vi "SCMP - Run Cookbook.vi"(0 "Cookbook":T13=[{"Data Type"=enum."SET EXPOSURE", "Arg 1"=0.1, "Arg 2"=999.0, "Arg 3"=path "C:/SCD Cookbooks/exposure-100ms.rcp", "Comments"=""}, {"Data Type"=enum."ACQUIRE DATA", "Arg 1"=1.0, "Arg 2"=1.0, "Arg 3"=path "C:/SCD Cookbooks/aaa.rcp", "Comments"=""}], 1 "Mod/Seq":bool, 3 "Save to FITS?":bool=TRUE, 5 "limit max FPS to:":dbl=20.0 format="%0.2p", 7 "Motors":bool=TRUE, 11 "Error in":errorcluster, 12 "Andor Neo":T1[](array[typedef]) {"Exposure (s)" format="%^.3g"; "Time at Synch" format="%<%H:%M:%S>T"; "Interframe Time" format="%#_3g"; "Frame Readout Time" format="%_3g"; "Row Readout Time" format="%_3g"}, 13 "FITS Header In":T4={"Wavelength (nm)"=530.15, "Exposure (s)"=0.05, "Tuning Delay (ms)"=1000.0, "Beam Type (-1/1)"=1.0, "Tuning Voltages"=[1.111, 2.222, 3.333, 4.444], "Observer"="observer", "Light Shapping Diffuser"=enum."In Beam", "Comment"="", "Data Type"=9, "Mod Cycles"=0, "SCD Calibration Optics"=enum."1 - Polarizer @0, I+Q", "SCD Emission Line Filter"=enum."1-557.6nm", "Cookbook"="", "COMP-S Calibration Wheel"=enum."Dark", "COMP-S Andover Filter Wheel"=enum."530.3nm/HWB 0.34nm (Fe XIV)", "FOV Rotation (deg)"=66.0, "Objective Lens Position (mm)"=0.0, "Occulter size"=0.0, "Time End"=timestamp(3382374145.421875 s since 1904-01-01), "Acc Exposure (s)"=0.0, "Time Stamp Array"=[], "Camera Serial Number"=[], "Camera Temp"=[], "Camera PI (mm)"=[], "Time Start"=timestamp(3382374145.421875 s since 1904-01-01), "Peripherals"={"ILX controler"=FALSE, "Zone temperatures"=FALSE, "Andor"=FALSE, "Andor 2"=FALSE, "PI Stages"=FALSE, "AISAS mechanisms"=FALSE, "AISAS Mech.lvclass"=refnum, "Zone temp ref"=variant, "FWs"=FALSE}, "FITS paths"=[], "Cameras"=enum."Andor", "load preset cbk"=FALSE, "periodic check count"=0} {"Camera PI (mm)" format="%_3g"; "Acc Exposure (s)" format="%^.3g"; "Occulter size" format="%.2f"; "Objective Lens Position (mm)" min=70.0 max=152.0 format="%.2f"; "FOV Rotation (deg)" format="%.1f"; "Data Type" items=["LIVE", "DARK", "FLAT", "CALI", "OBSE", "ABSO", "AURE", "TARG", "OBJE", "HOLE", "OREX", "THRO", "CHIP"]; "Exposure (s)" format="%^.3g"; "Wavelength (nm)" format="%_6g"}) -> (4 "Result":string, 6 "FITS Path Out":path, 14 "Updated Header":T4={"Wavelength (nm)"=530.15, "Exposure (s)"=0.05, "Tuning Delay (ms)"=1000.0, "Beam Type (-1/1)"=1.0, "Tuning Voltages"=[1.111, 2.222, 3.333, 4.444], "Observer"="observer", "Light Shapping Diffuser"=enum."In Beam", "Comment"="", "Data Type"=9, "Mod Cycles"=0, "SCD Calibration Optics"=enum."1 - Polarizer @0, I+Q", "SCD Emission Line Filter"=enum."1-557.6nm", "Cookbook"="", "COMP-S Calibration Wheel"=enum."Dark", "COMP-S Andover Filter Wheel"=enum."530.3nm/HWB 0.34nm (Fe XIV)", "FOV Rotation (deg)"=66.0, "Objective Lens Position (mm)"=0.0, "Occulter size"=0.0, "Time End"=timestamp(3382374145.421875 s since 1904-01-01), "Acc Exposure (s)"=0.0, "Time Stamp Array"=[], "Camera Serial Number"=[], "Camera Temp"=[], "Camera PI (mm)"=[], "Time Start"=timestamp(3382374145.421875 s since 1904-01-01), "Peripherals"={"ILX controler"=FALSE, "Zone temperatures"=FALSE, "Andor"=FALSE, "Andor 2"=FALSE, "PI Stages"=FALSE, "AISAS mechanisms"=FALSE, "AISAS Mech.lvclass"=refnum, "Zone temp ref"=variant, "FWs"=FALSE}, "FITS paths"=[], "Cameras"=enum."Andor", "load preset cbk"=FALSE, "periodic check count"=0} {"Camera PI (mm)" format="%_3g"; "Acc Exposure (s)" format="%^.3g"; "Occulter size" format="%.2f"; "Objective Lens Position (mm)" min=70.0 max=152.0 format="%.2f"; "FOV Rotation (deg)" format="%.1f"; "Data Type" items=["LIVE", "DARK", "FLAT", "CALI", "OBSE", "ABSO", "AURE", "TARG", "OBJE", "HOLE", "OREX", "THRO", "CHIP"]; "Exposure (s)" format="%^.3g"; "Wavelength (nm)" format="%_6g"}, 15 "Error out":errorcluster)   [LabVIEW 2014]
doc: "Use this template to build a VI to use as a subVI."
uses:
  Controls/Cookbook.ctl
  Controls/Cbk Data type.ctl
  Controls/SCD - FITS Cluster.ctl
  AISAS/Mech/AISAS Mech.lvclass
  AISAS/Controls/Diffuser.ctl
  Controls/SCD - Calibration Optics Filter Wheel.ctl
  Controls/SCD - EDT - Emission Line Filter Wheel.ctl
  Controls/CoMP-S Controls/Polarization Optics Filter Wheel.ctl
  Controls/CoMP-S Controls/Emission Line Filter Wheel.ctl
  AISAS/Controls/focus.ctl
  Controls/peripherals.ctl
  Controls/Cameras select.ctl
  Camera/Andor Neo Info.ctl
  Controls/beaning.ctl
  AISAS/Controls/motor.ctl
  AISAS/Mech/AISAS Mech.lvclass/AISAS Mech.ctl
  Controls/Globals.vi
  <vilib>/Utility/file.llb/Read From Spreadsheet File (DBL).vi
panel:
  out "Changes 0 or 1 to true/false for absolute or relative control 4":bool[](array[boolean])
  out "Changes 0 or 1 to true/false for absolute or relative control 3":bool[](array[boolean])
  out "rcp first row":dbl[](array[numeric]) format="%0.4f"
  out "Changes 0 or 1 to true/false for absolute or relative control 2":bool[](array[boolean])
  in  "Stop Cookbook":bool
  out "Recipe Being Processed":string
  out "Most Recent Image Accumulation (Modulation State A)":u32[][](graph)
  out "Headers Out":T4[](array[typedef]) {"Camera PI (mm)" format="%_3g"; "Acc Exposure (s)" format="%^.3g"; "Occulter size" format="%.2f"; "Objective Lens Position (mm)" min=70.0 max=152.0 format="%.2f"; "FOV Rotation (deg)" format="%.1f"; "Data Type" items=["LIVE", "DARK", "FLAT", "CALI", "OBSE", "ABSO", "AURE", "TARG", "OBJE", "HOLE", "OREX", "THRO", "CHIP"]; "Exposure (s)" format="%^.3g"; "Wavelength (nm)" format="%_6g"}
  out "LCVR Voltages":dbl[][](array[numeric]) format="%.4f"
  out "Total Recipes":i32=2
  out "Recipe Step":i32=1
  out "Mod Cycles":u16=1
  out "Exposure (s)":sgl=0.1
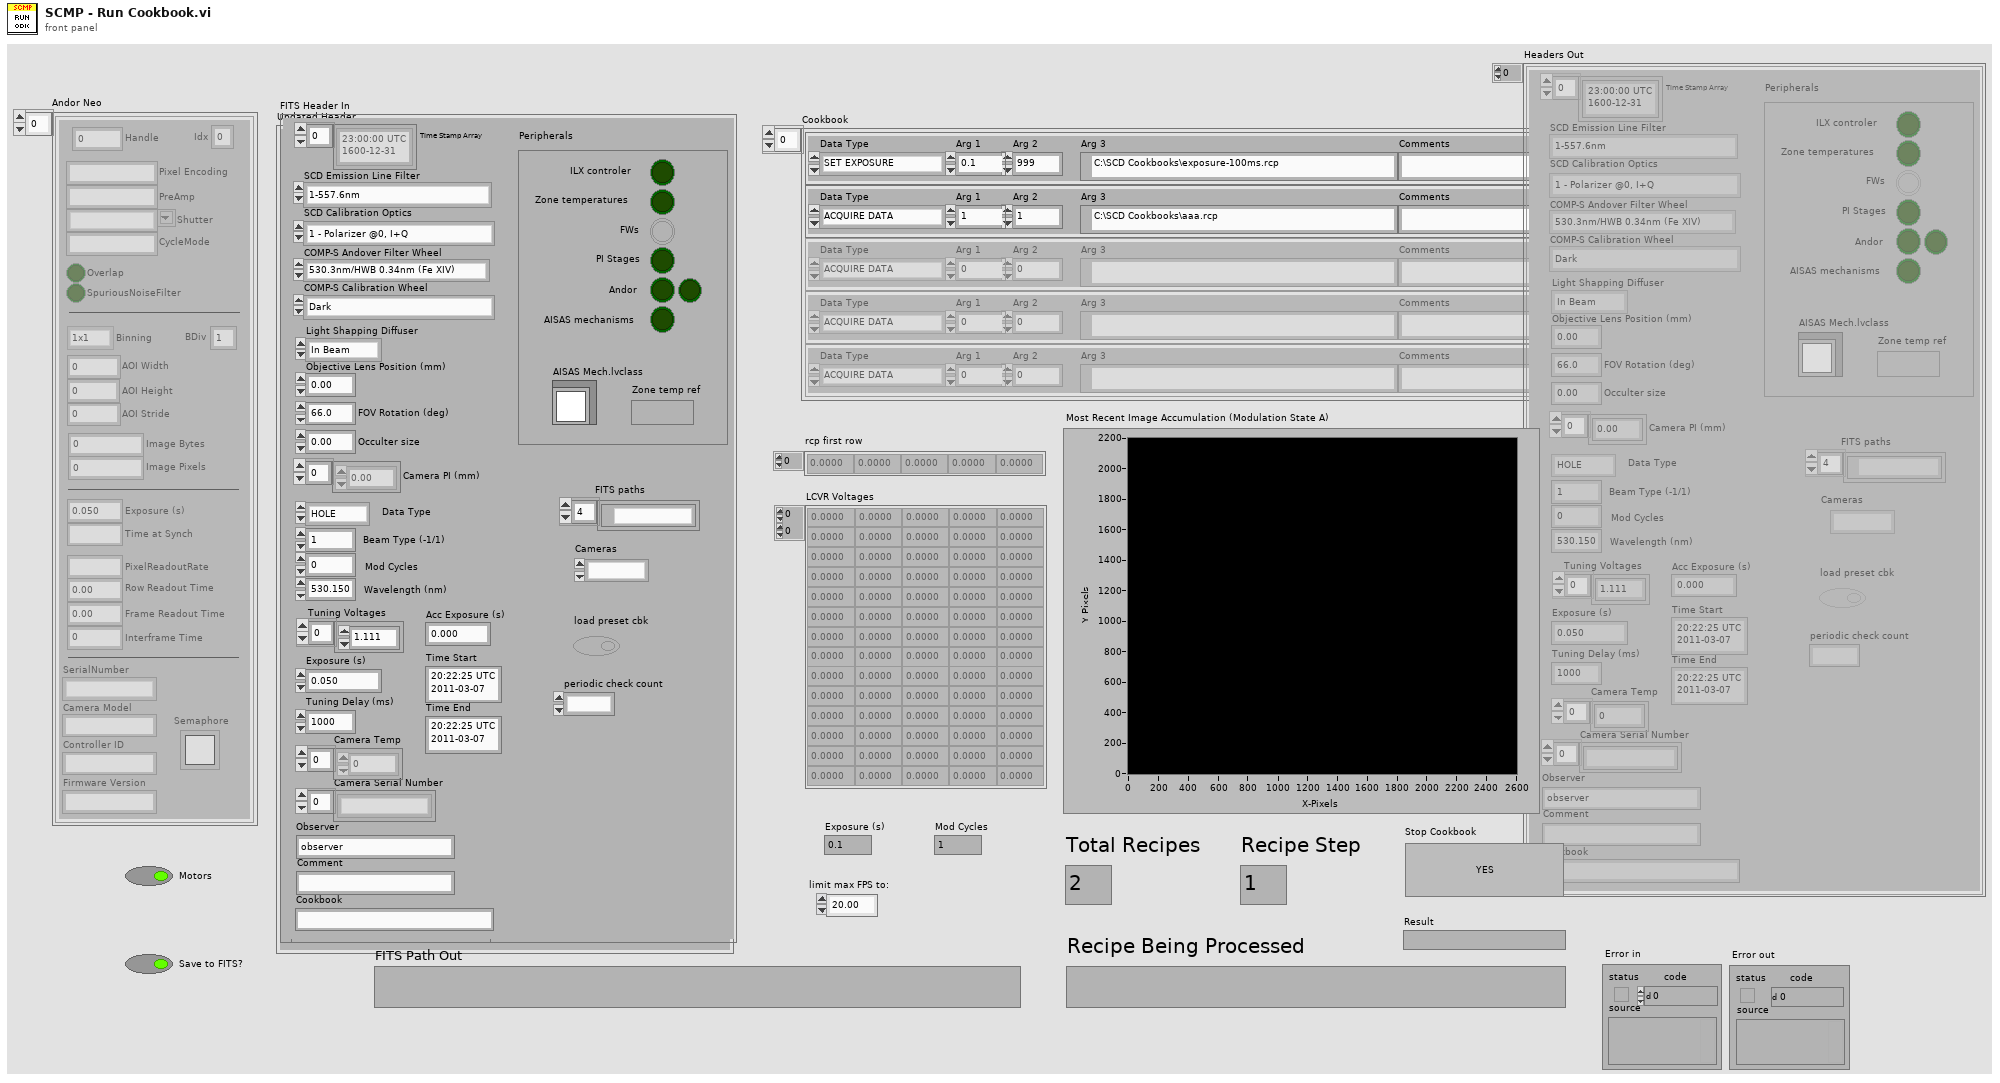
[diagram p1: front panel]
types:
  T1 = typedef "Andor Neo Info.ctl" = cluster{"Handle":i32, "Pixel Encoding":string, "AOI Width":i32, "AOI Height":i32, "AOI Stride":i32, "Row Readout Time":dbl, "Frame Readout Time":dbl, "Interframe Time":dbl, "Semaphore":T2, "SerialNumber":string, "Camera Model":string, "Controller ID":string, "Firmware Version":string, "Shutter":string, "BDiv":u8, "Time at Synch":timestamp, "Idx":i32, "PreAmp":string, "Binning":T3, "PixelReadoutRate":string, "Exposure (s)":dbl, "Image Bytes":i64, "Image Pixels":i64, "SpuriousNoiseFilter":bool, "Overlap":bool, "CycleMode":string}
  T2 = typedef "Semaphore RefNum" = refnum<k1>
  T3 = typedef "beaning.ctl" = enum16{"1x1", "2x2", "3x3", "4x4", "8x8"}
  T4 = typedef "SCD - FITS Cluster.ctl" = cluster{"Wavelength (nm)":dbl, "Exposure (s)":dbl, "Tuning Delay (ms)":dbl, "Beam Type (-1/1)":dbl, "Tuning Voltages":dbl[], "Observer":string, "Light Shapping Diffuser":T5, "Comment":string, "Data Type":u16, "Mod Cycles":u16, "SCD Calibration Optics":T6, "SCD Emission Line Filter":T7, "Cookbook":string, "COMP-S Calibration Wheel":T8, "COMP-S Andover Filter Wheel":T9, "FOV Rotation (deg)":dbl, "Objective Lens Position (mm)":T10, "Occulter size":dbl, "Time End":timestamp, "Acc Exposure (s)":dbl, "Time Stamp Array":timestamp[], "Camera Serial Number":string[], "Camera Temp":dbl[], "Camera PI (mm)":dbl[], "Time Start":timestamp, "Peripherals":T11, "FITS paths":path[], "Cameras":T12, "load preset cbk":bool, "periodic check count":i32}
  T5 = typedef "Diffuser.ctl" = enum16{"Out of Beam", "In Beam"}
  T6 = typedef "SCD - Calibration Optics Filter Wheel.ctl" = enum16{"1 - Polarizer @0, I+Q", "2 - Polarizer @90, I-Q", "3 - Polarizer @45, I+U", "4 - Polarizer @135, I-U", "5 - Polarizer @0, Retarder @45, I+V", "6 - Polarizer @0, Retarder @135, I-V", "7 - Dark", "8 - Clear", "9 - N/A"}
  T7 = typedef "SCD - EDT - Emission Line Filter Wheel.ctl" = enum16{"1-557.6nm", "2-587.6nm", "3-589.6nm", "4-630.2nm", "5-656.4nm", "6-849.8nm", "7-854.2nm", "8-866.2nm", "9-1083.0nm"}
  T8 = typedef "Polarization Optics Filter Wheel.ctl" = enum16{"Dark", "Clear", "Exchange Lens", "Polarizer @0, I+Q", "Polarizer @90, I-Q", "Polarizer @45, I+U", "Polarizer @135, I-U", "Polarizer @0, Retarder @45, I+V", "Polarizer @0, Retarder @135, I-V"}
  T9 = typedef "Emission Line Filter Wheel.ctl" = enum16{"530.3nm/HWB 0.34nm (Fe XIV)", "587.6nm/HBW 0.44nm (He I D3)", "637.5nm/HBW 0.53nm (Fe X)", "656.3nm/HBW 0.57nm (H-Alpha)", "789.2nm/HBW 0.85nm (Fe XI)", "854.2nm/HBW 1.01nm (Ca I)", "1074.7nm/HBW 2.34nm (Fe XIII)", "1079.8nm/HBW 1.64nm (Fe XIII)", "1083.0nm/HBW 1.66nm (He I)"}
  T10 = typedef "focus.ctl" = dbl
  T11 = typedef "peripherals.ctl" = cluster{"ILX controler":bool, "Zone temperatures":bool, "Andor":bool, "Andor 2":bool, "PI Stages":bool, "AISAS mechanisms":bool, "AISAS Mech.lvclass":refnum<class "AISAS Mech.lvclass">, "Zone temp ref":variant, "FWs":bool}
  T12 = typedef "Cameras select.ctl" = enum16{"Andor", "GDR"}
  T13 = typedef "Cookbook.ctl" = cluster{"Data Type":T14, "Arg 1":sgl, "Arg 2":sgl, "Arg 3":path, "Comments":string}[]
  T14 = typedef "Cbk Data type.ctl" = enum32{"ACQUIRE DATA", "SET DIFFUSER", "CAL-FW", "WAVELENGTH-FW", "INSTR. ROTATION", "SET FOCUS", "DATATYPE", "SET EXPOSURE", "CBK COMMENTS", "MOVE-PI", "MOVE-PI2", "MOVE-PI3", "DWELL TIME", "BINNING"}
  T15 = typedef "motor.ctl" = enum32{"Rotation", "Diffuser ", "Focus"}
  T16 = enum16{"Emission Line Filters", "Calibration Polarizers"}
  T17 = typedef "Rotation.ctl" = dbl
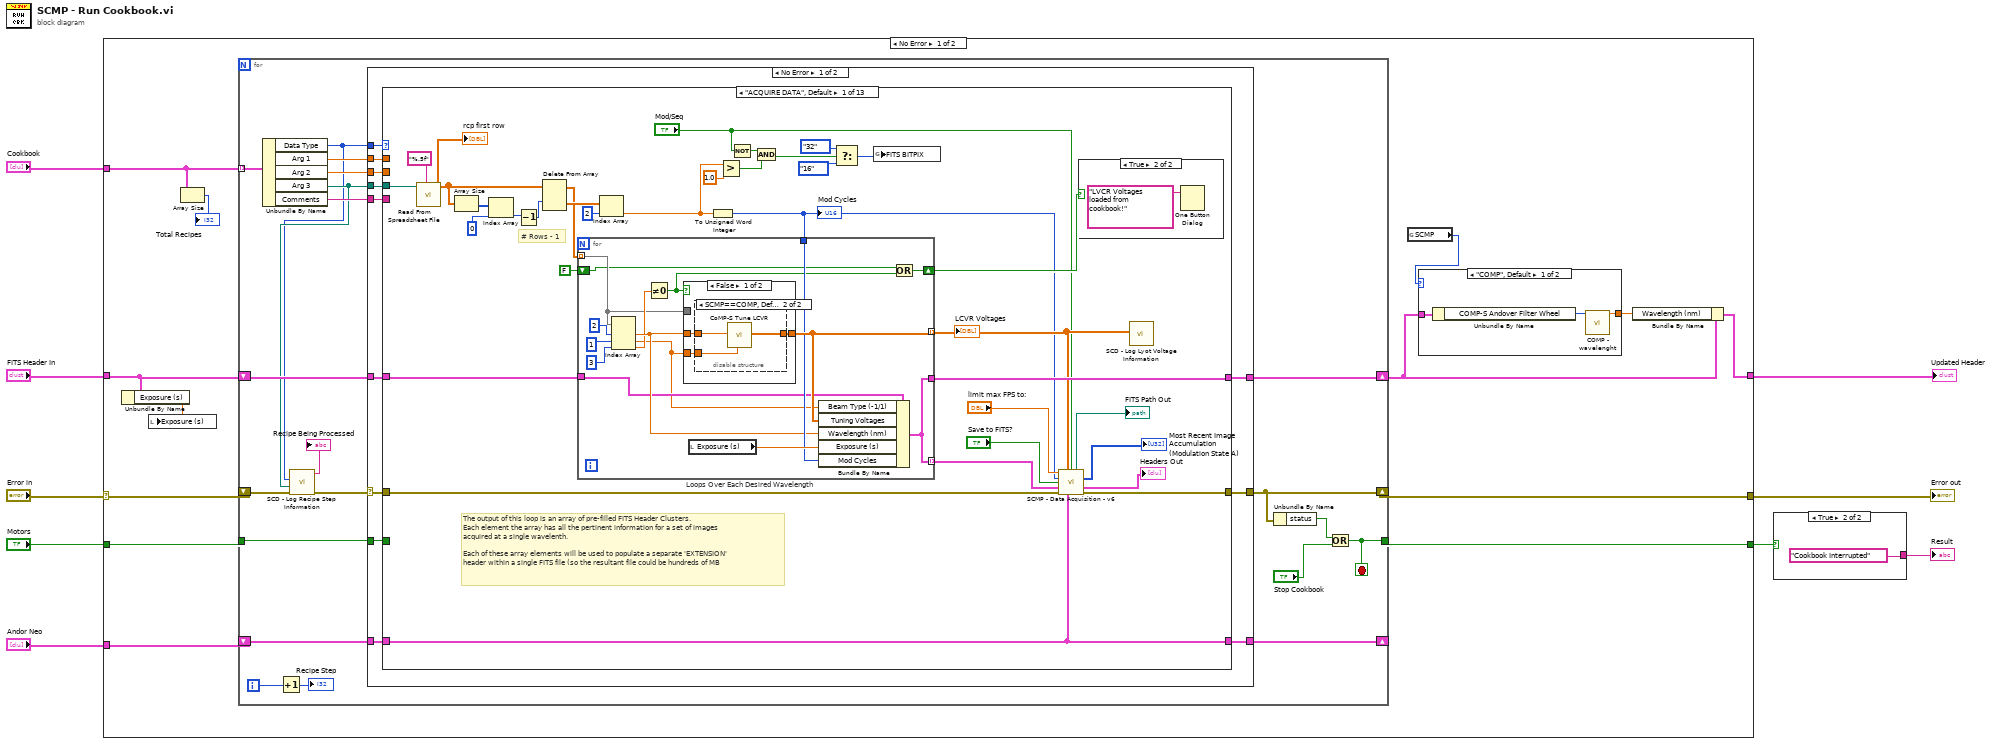
[diagram p0: block diagram]
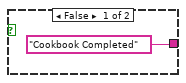
[diagram p2: hidden frame]
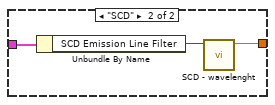
[diagram p3: hidden frame]
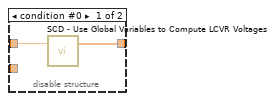
[diagram p5: hidden frame]
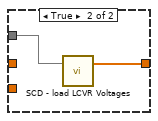
[diagram p6: hidden frame]
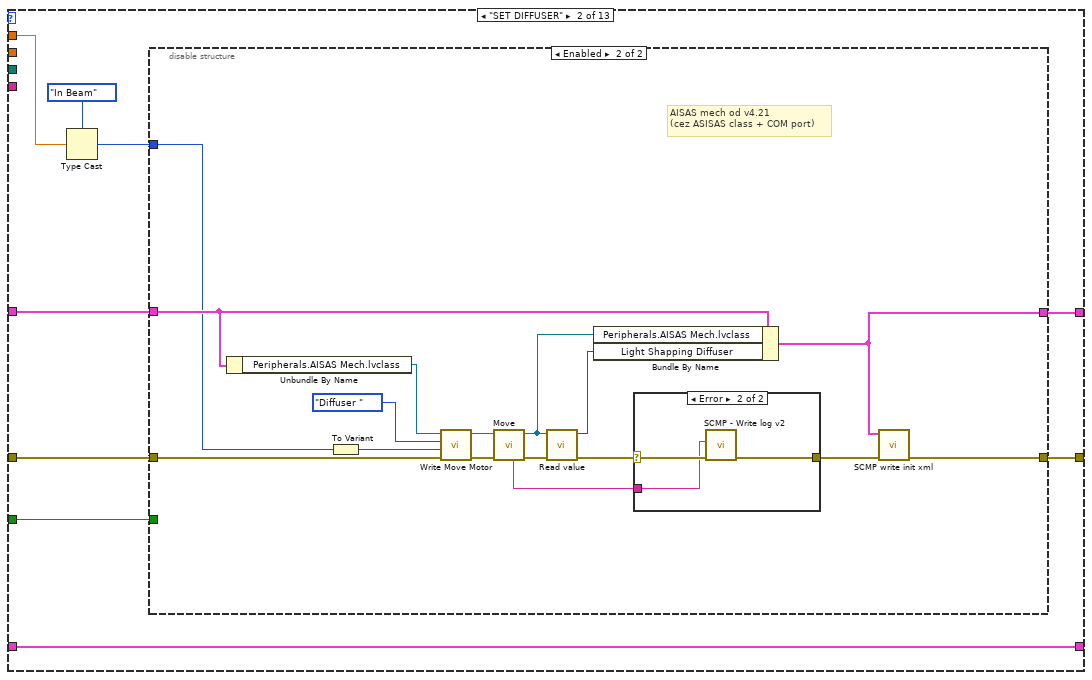
[diagram p7: hidden frame]
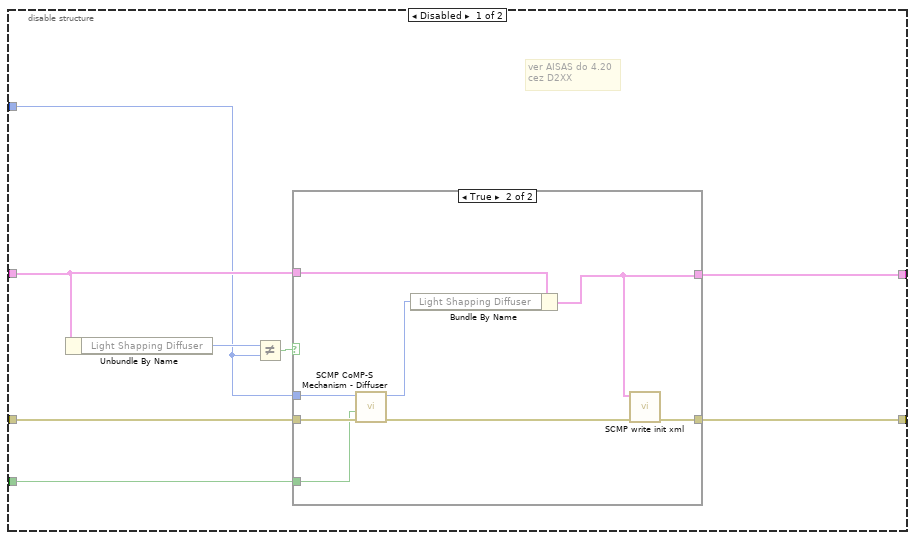
[diagram p8: hidden frame]
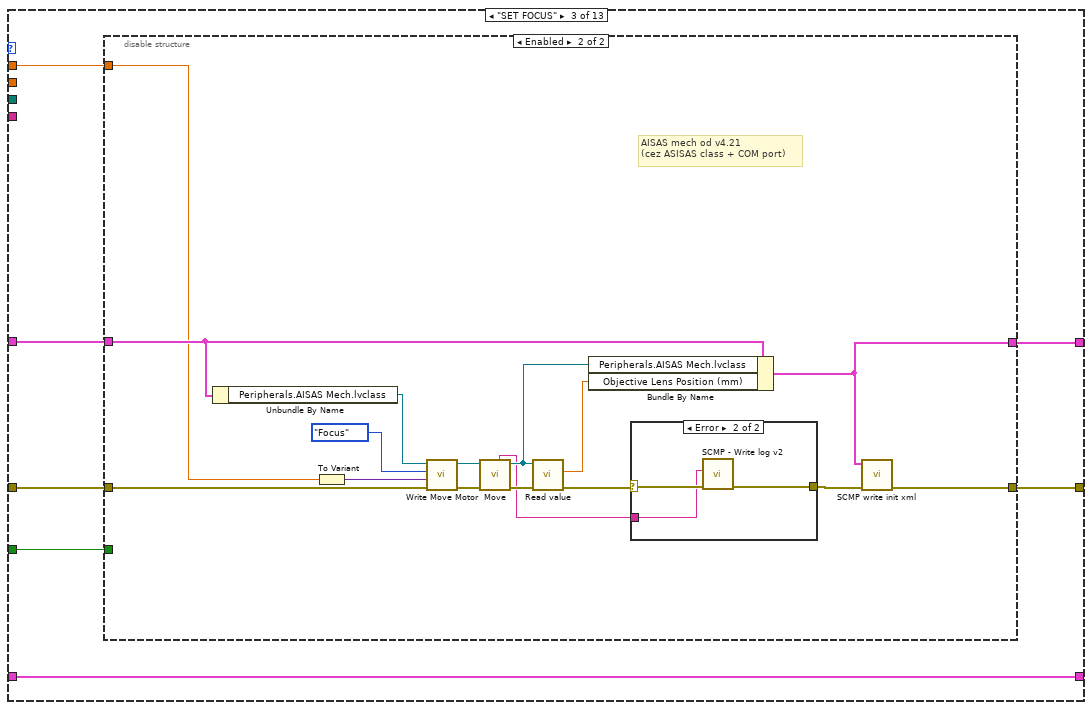
[diagram p11: hidden frame]
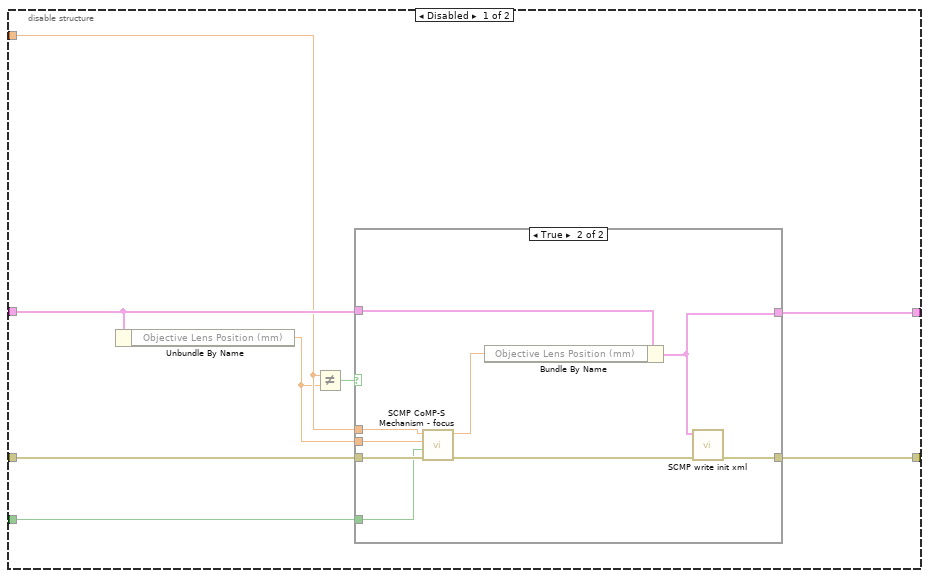
[diagram p12: hidden frame]
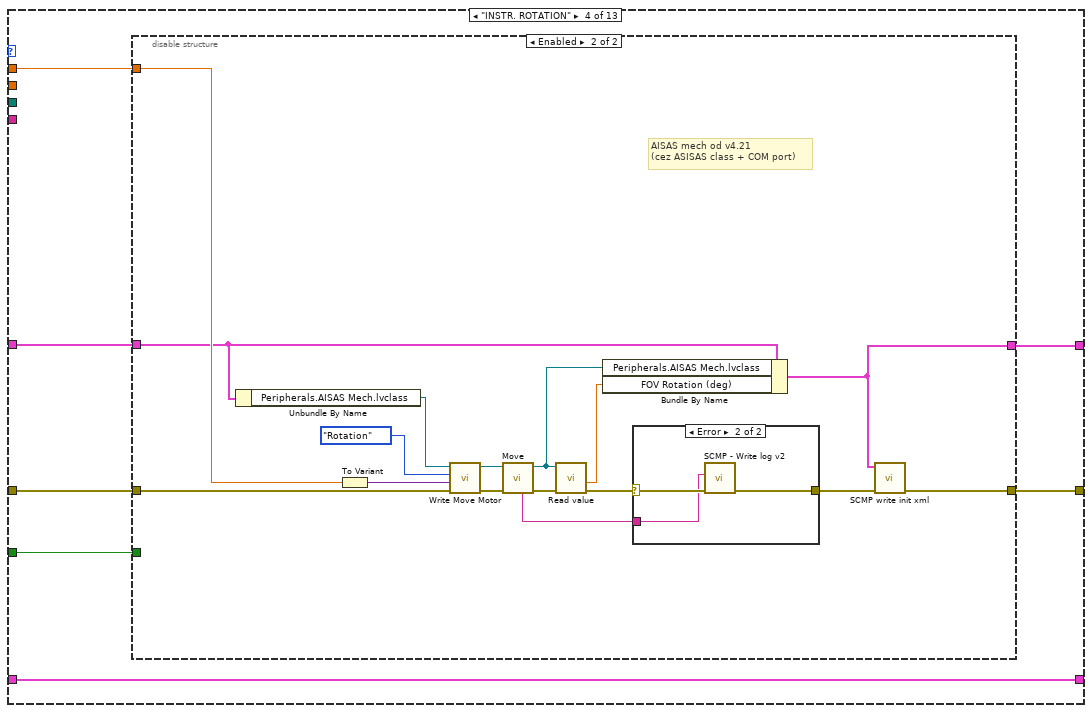
[diagram p15: hidden frame]
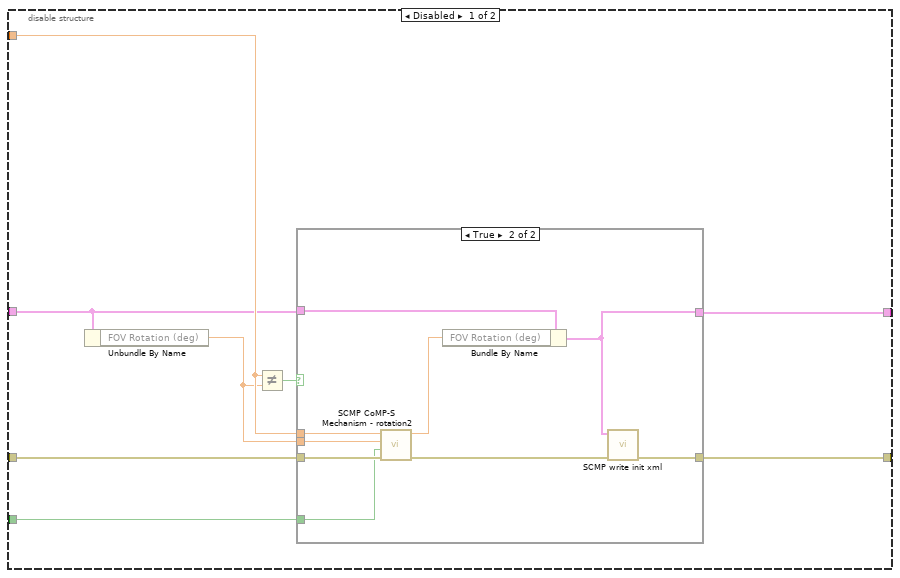
[diagram p16: hidden frame]
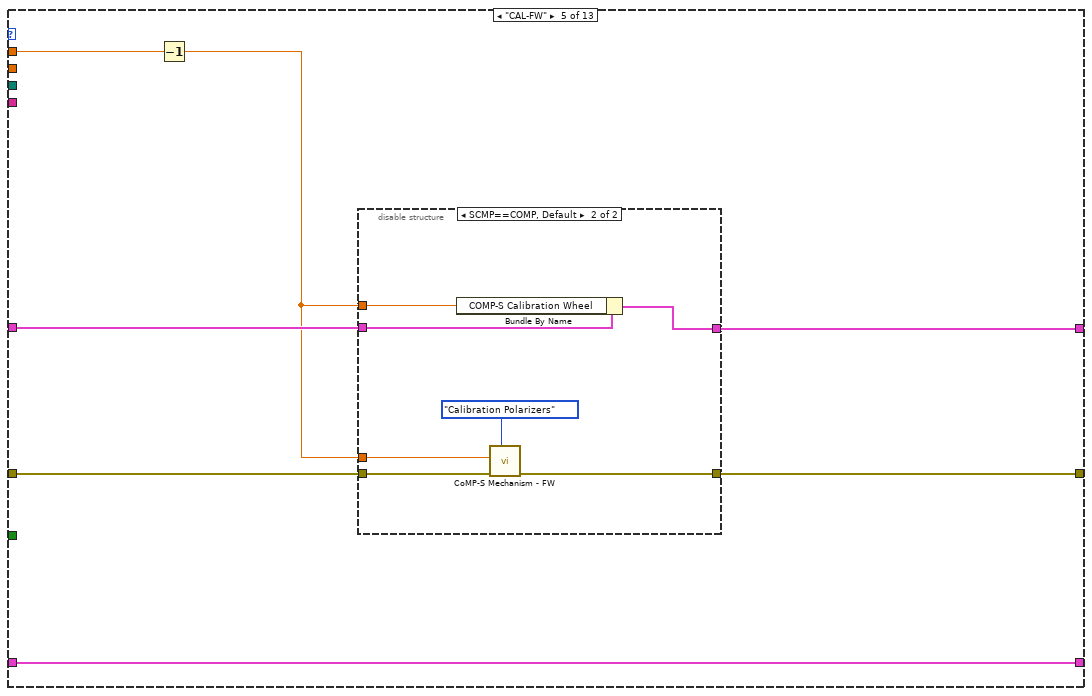
[diagram p19: hidden frame]
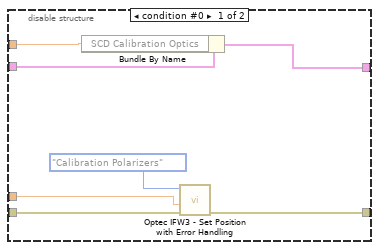
[diagram p20: hidden frame]
diagram:
  n1 = case shown="No Error" "Error in" {
    selector: "Error in" -> [w19 w429]
    tunnel: [w21 w429] -> w8
    tunnel: [w18 TRUE] -> w6
    tunnel: "FITS Header In" -> [w17 w427]
    tunnel: "Cookbook" -> [w16 _]
    tunnel: "Motors" -> [w15 _]
    tunnel: "Andor Neo" -> [w14 _]
    tunnel: [w12 w427] -> w1
    frame No Error {
      n2 = Unbundle By Name(w17) -> ("Exposure (s)"=w20:dbl)
      n3 = local write "Exposure (s)"(w20) -> ()
      n4 = Array Size(array=w16) -> (size(s)=→"Total Recipes":i32)
      n5 = for {
        tunnel: w16 -> [w44] mode=indexing
        shift-right: [w38] -> w13
        shift-left: w17 -> [w45]
        shift-right: [w30] -> w21
        shift-left: w19 -> [w41]
        tunnel: w15 -> [w35]
        shift-right: [w33] -> _
        shift-left: w14 -> [w34]
        tunnel: [w29] -> w18
        i -> [w40]
        stop <- w29 stop-if-true
        n6 = Unbundle By Name(w44) -> ("Data Type"=w37:T14, "Arg 1"=w47:sgl, "Arg 2"=w48:sgl, "Arg 3"=w43:path, "Comments"=w46:string)
        n7 = Increment(x=w40) -> (x+1=→"Recipe Step":i32)
        n8 = call "SCD - Log Recipe Step Information.vi"("error in (no error)"=w41, "Arg 3"=w43, "Data Type"=w37) -> ("error out"=w36:errorcluster, "Recipe Being Processed"=→"Recipe Being Processed":string)  [unwired: 7 in]
        n9 = case shown="No Error" w36 {
          selector: w36 -> [w52 w425]
          tunnel: w48 -> [w60 _]
          tunnel: w37 -> [w59 _]
          tunnel: w47 -> [w58 _]
          tunnel: w43 -> [w57 _]
          tunnel: w46 -> [w56 _]
          tunnel: w45 -> [w55 w426]
          tunnel: [w54 w426] -> w38
          tunnel: [w53 w425] -> w30
          tunnel: w35 -> [w51 _]
          tunnel: w34 -> [w50 w424]
          tunnel: [w49 w424] -> w33
          frame No Error {
            n10 = case shown="\"ACQUIRE DATA\", Default" w59 {
              tunnel: w60 -> [_ _ _ _ _ _ _ _ _ w350 w372 w394 _]
              tunnel: w58 -> [_ w126 w169 w215 w263 w284 w305 w330 _ w353 w375 w397 w416]
              tunnel: w57 -> [w95 _ _ _ _ _ _ _ _ _ _ _ _]
              tunnel: w52 -> [w82 w128 w175 w220 w265 w286 w308 w328 w346 w351 w373 w395 w417]
              tunnel: [w85 w127 w174 w219 w264 w285 w308 w327 w345 w352 w374 w396 w413] -> w53
              tunnel: w56 -> [_ _ _ _ _ _ _ _ w344 _ _ _ _]
              tunnel: w55 -> [w86 w129 w172 w221 w266 w288 w307 w332 w343 w348 w370 w392 w418]
              tunnel: [w87 w130 w173 w218 w267 w287 w306 w331 w343 w354 w376 w398 w418] -> w54
              tunnel: w51 -> [_ w123 w171 w217 _ _ _ _ _ _ _ _ _]
              tunnel: w50 -> [w61 w122 w170 w216 w261 w282 w303 w324 w342 w349 w371 w393 w419]
              tunnel: [w61 w122 w170 w216 w261 w282 w303 w323 w342 w349 w371 w393 w419] -> w49
              frame "ACQUIRE DATA", Default {
                # "The output of this loop is an array of pre-filled FITS Header Clusters.\nEach element the array has all the pertinent information for a set of images\nacquired at a single wavelenth.\n\nEach of these array elements will be used to populate a separate 'EXTENSION'\nheader within a single FITS file (so the resultant file could be hundreds of MB"
                # "# Rows - 1"
                n11 = call-poly <vilib>:"Read From Spreadsheet File.vi"("format (%.3f)"="%.5f", "file path (dialog if empty)"=w95) -> ("first row"=→"rcp first row":dbl[], "all rows"=w94:dbl[][])  [unwired: 5 in, 3 out]
                n12 = Array Size(array=w94) -> (size(s)=w93:i32[])
                n13 = Index Array(array=w93, index=0) -> (element=w92:i32)
                n14 = Decrement(x=w92) -> (x-1=w91:i32)
                n15 = Delete From Array "Delete From Array"(array=w94, index (row)=w91) -> (deleted portion=w90:dbl[], array with subset deleted=w88:dbl[][])  [unwired: 2 in]
                n16 = Index Array(array=w90, index=2) -> (element=w67:dbl)
                n17 = To Unsigned Word Integer(number=w67) -> (unsigned 16bit integer=w68:u16)
                "Mod Cycles" <- w68
                n18 = for "Loops Over Each Desired Wavelength" {
                  tunnel: w88 -> [w101] mode=indexing
                  tunnel: [w107] -> w84 mode=indexing
                  tunnel: [w108] -> w83 mode=indexing
                  tunnel: w86 -> [w103]
                  tunnel: [w108] -> w87
                  tunnel: w68 -> [w106]
                  shift-right: [w100] -> w79
                  shift-left: FALSE -> [w99]
                  n19 = Index Array(array=w101, index #1=2 ("index"), index #2=1 ("index"), index #3=3 ("index")) -> (element #1=w105:dbl, element #2=w97:dbl, element #3=w102:dbl)
                  n20 = Not Equal To 0?(x=w102) -> (x != 0?=w98:bool)
                  n21 = case shown="False" w98 {
                    tunnel: [w114 w121] -> w107
                    tunnel: w105 -> [w113 _]
                    tunnel: w101 -> [_ w120]
                    tunnel: w97 -> [w112 _]
                    frame False {
                      n22 = disable-structure shown="SCMP==COMP, Default" {
                        disable-tunnel: [w116 w119] -> w114
                        disable-tunnel: w113 -> [w115 w118]
                        disable-tunnel: w112 -> [_ w117]
                        frame condition #0 {
                          n23 = call "SCD - Use Global Variables to Compute LCVR Voltages.vi"("Wavelength (nm)"=w115) -> ("Required LCVR Voltages"=w116:dbl[])  [unwired: 1 in, 1 out]
                        }
                        frame condition #1 (active) {
                          n24 = call "CoMP-S Tune LCVR.vi"("Beam"=w117, "Wavelength (nm)"=w118) -> ("Required LCVR Voltages"=w119:dbl[])  [unwired: 8 in, 1 out]
                        }
                      }
                    }
                    frame True {
                      n25 = call "SCD - load LCVR Voltages.vi"("input rcp"=w120) -> ("Required LCVR Voltages"=w121:dbl[])  [unwired: 2 in]
                    }
                  }
                  n26 = local read "Exposure (s)"() -> (w109:sgl)
                  n27 = Bundle By Name(cluster=w103, "Beam Type (-1/1)"=w97, "Tuning Voltages"=w107, "Wavelength (nm)"=w105, "Exposure (s)"=w109, "Mod Cycles"=w106) -> (w108:T4)
                  n28 = Or(x=w99, y=w98) -> (x .or. y?=w100:bool)
                }
                "LCVR Voltages" <- w84
                n29 = Greater?(x=w67, y=1.0) -> (0:w64:bool)
                n30 = Not(x="Mod/Seq") -> (.not. x?=w63:bool)
                n31 = And(x=w63, y=w64) -> (x .and. y?=w65:bool)
                n32 = Select(t=enum16{"16", "32"}."32" ("FITS BITPIX"), s=w65, f=enum16{"16", "32"}."16") -> (s? t:f=w71:enum16{"16", "32"})
                n33 = global write "Globals.vi" "FITS BITPIX"(w71) -> ()
                n34 = call "SCMP - Data Acquisition - v6.vi"("Max FPS limit"="limit max FPS to:", "LCVR Voltages"=w84, "Mod/Seq"="Mod/Seq", "Cycles"=w68, "Save to FITS?"="Save to FITS?", "Headers In"=w83, "error in"=w82, "Andor Neo"=w61) -> ("FITS Path Out"=→"FITS Path Out":path, "Image"=→"Most Recent Image Accumulation (Modulation State A)":u32[][], "Headers Out"=→"Headers Out":T4[], "error out"=w85:errorcluster)  [unwired: 2 in, 2 out]
                n35 = case shown="True" w79 {
                  frame False {
                  }
                  frame True {
                    n36 = One Button Dialog(message="LVCR Voltages loaded from cookbook!") -> ()  [unwired: 1 in, 1 out]
                  }
                }
                n37 = call "SCD - Log Lyot Voltage Information.vi"("array"=w84) -> ()  [unwired: 10 in, 1 out]
              }
              frame "SET DIFFUSER" {
                n38 = Type Cast(type=Diffuser."In Beam" ("Light Shapping Diffuser"), x=w126) -> (*(type *) &x=w124:T5)
                n39 = disable-structure shown="Enabled" {
                  disable-tunnel: [w138 w153] -> w130
                  disable-tunnel: w129 -> [w137 w161]
                  disable-tunnel: w128 -> [w135 w160]
                  disable-tunnel: [w134 w154] -> w127
                  disable-tunnel: w124 -> [w132 w159]
                  disable-tunnel: w123 -> [w131 _]
                  frame Disabled {
                    # "ver AISAS do 4.20\ncez D2XX"
                    n40 = Unbundle By Name(w137) -> ("Light Shapping Diffuser"=w133:T5)
                    n41 = Not Equal?(x=w133, y=w132) -> (x != y?=w136:bool)
                    n42 = case shown="True" w136 {
                      tunnel: [w140 w141] -> w138
                      tunnel: w137 -> [w140 w145]
                      tunnel: w135 -> [w139 w147]
                      tunnel: [w139 w148] -> w134
                      tunnel: w132 -> [_ w144]
                      tunnel: w131 -> [_ w143]
                      frame False {
                        # "mh: generovat warning ze cbk reduntantne nastavuje difuser?"
                      }
                      frame True {
                        n43 = call "SCMP CoMP-S Mechanism - Diffuser.vi"("error in (no error)"=w147, "Auto Motors"=w143, "Desired Diffuser"=w144) -> ("error out"=w146:errorcluster, "New Diffuser"=w142:T5)  [unwired: 7 in]
                        n44 = Bundle By Name(cluster=w145, "Light Shapping Diffuser"=w142) -> (w141:T4)
                        n45 = call "SCMP write init xml.vi"("error in (no error)"=w146, "FITS Header In"=w141) -> ("error out"=w148:errorcluster)  [unwired: 8 in, 1 out]
                      }
                    }
                  }
                  frame Enabled {
                    # "AISAS mech od v4.21\n(cez ASISAS class + COM port)"
                    n46 = Unbundle By Name(w161) -> ("Peripherals.AISAS Mech.lvclass"=w164:refnum<class "AISAS Mech.lvclass">)
                    n47 = To Variant(anything=w159) -> (Variant=w163:variant)
                    n48 = call "Write Move Motor.vi"("error in (no error)"=w160, "Desired Value"=w163, "Motor"=motor."Diffuser ", "AISAS Mech in"=w164) -> ("error out"=w157:errorcluster, "AISAS Mech out"=w156:refnum<class "AISAS Mech.lvclass">)  [unwired: 6 in]
                    n49 = call "Move.vi"("error in (no error)"=w157, "AISAS Mech in"=w156) -> ("error out"=w158:errorcluster, "AISAS Mech out"=w152:refnum<class "AISAS Mech.lvclass">, "status log"=w149:string)  [unwired: 7 in]
                    n50 = call "Read value.vi"("error in (no error)"=w158, "AISAS Mech in"=w152) -> ("error out"=w151:errorcluster, "Diffuser"=w155:T5)  [unwired: 3 in, 5 out]
                    n51 = Bundle By Name(cluster=w161, "Peripherals.AISAS Mech.lvclass"=w152, "Light Shapping Diffuser"=w155) -> (w153:T4)
                    n52 = case shown="Error" w151 {
                      selector: w151 -> [w165 w168]
                      tunnel: [w165 w167] -> w150
                      tunnel: w149 -> [_ w166]
                      frame No Error {
                      }
                      frame Error {
                        n53 = call "SCMP - Write log v2.vi"("Error to log"=w168, "data"=w166) -> ("error out"=w167:errorcluster)  [unwired: 7 in, 2 out]
                      }
                    }
                    n54 = call "SCMP write init xml.vi"("error in (no error)"=w150, "FITS Header In"=w153) -> ("error out"=w154:errorcluster)  [unwired: 8 in, 1 out]
                  }
                }
              }
              frame "SET FOCUS" {
                n55 = disable-structure shown="Enabled" {
                  disable-tunnel: w175 -> [w183 w200]
                  disable-tunnel: [w182 w201] -> w174
                  disable-tunnel: [w181 w202] -> w173
                  disable-tunnel: w172 -> [w179 w203]
                  disable-tunnel: w169 -> [w178 w199]
                  disable-tunnel: w171 -> [w176 _]
                  frame Disabled {
                    n56 = Unbundle By Name(w179) -> ("Objective Lens Position (mm)"=w177:T10)
                    n57 = Not Equal?(x=w178, y=w177) -> (x != y?=w180:bool)
                    n58 = case shown="True" w180 {
                      tunnel: [w185 w186] -> w181
                      tunnel: w179 -> [w185 w192]
                      tunnel: w183 -> [w184 w191]
                      tunnel: [w184 w194] -> w182
                      tunnel: w178 -> [_ w190]
                      tunnel: w177 -> [_ w189]
                      tunnel: w176 -> [_ w188]
                      frame False {
                        # "mh: generovat warning ze cbk nastavuje reduntantne ?"
                      }
                      frame True {
                        n59 = call "SCMP CoMP-S Mechanism - focus.vi"("error in (no error)"=w191, "Auto Motors"=w188, "Old Focus"=w189, "Desired Focus"=w190) -> ("error out"=w193:errorcluster, "Focus out"=w187:dbl)  [unwired: 6 in]
                        n60 = Bundle By Name(cluster=w192, "Objective Lens Position (mm)"=w187) -> (w186:T4)
                        n61 = call "SCMP write init xml.vi"("error in (no error)"=w193, "FITS Header In"=w186) -> ("error out"=w194:errorcluster)  [unwired: 8 in, 1 out]
                      }
                    }
                  }
                  frame Enabled {
                    # "AISAS mech od v4.21\n(cez ASISAS class + COM port)"
                    n62 = Unbundle By Name(w203) -> ("Peripherals.AISAS Mech.lvclass"=w210:refnum<class "AISAS Mech.lvclass">)
                    n63 = To Variant(anything=w199) -> (Variant=w209:variant)
                    n64 = call "Write Move Motor.vi"("error in (no error)"=w200, "Desired Value"=w209, "Motor"=motor."Focus", "AISAS Mech in"=w210) -> ("error out"=w206:errorcluster, "AISAS Mech out"=w205:refnum<class "AISAS Mech.lvclass">)  [unwired: 6 in]
                    n65 = call "Move.vi"("error in (no error)"=w206, "AISAS Mech in"=w205) -> ("error out"=w207:errorcluster, "AISAS Mech out"=w204:refnum<class "AISAS Mech.lvclass">, "status log"=w195:string)  [unwired: 7 in]
                    n66 = call "Read value.vi"("error in (no error)"=w207, "AISAS Mech in"=w204) -> ("error out"=w197:errorcluster, "Focus"=w198:T10)  [unwired: 3 in, 5 out]
                    n67 = Bundle By Name(cluster=w203, "Peripherals.AISAS Mech.lvclass"=w204, "Objective Lens Position (mm)"=w198) -> (w202:T4)
                    n68 = case shown="Error" w197 {
                      selector: w197 -> [w211 w214]
                      tunnel: [w211 w213] -> w196
                      tunnel: w195 -> [_ w212]
                      frame No Error {
                      }
                      frame Error {
                        n69 = call "SCMP - Write log v2.vi"("Error to log"=w214, "data"=w212) -> ("error out"=w213:errorcluster)  [unwired: 7 in, 2 out]
                      }
                    }
                    n70 = call "SCMP write init xml.vi"("error in (no error)"=w196, "FITS Header In"=w202) -> ("error out"=w201:errorcluster)  [unwired: 8 in, 1 out]
                  }
                }
              }
              frame "INSTR. ROTATION" {
                n71 = disable-structure shown="Enabled" {
                  disable-tunnel: w215 -> [w228 w249]
                  disable-tunnel: w221 -> [w226 w248]
                  disable-tunnel: w220 -> [w225 w247]
                  disable-tunnel: [w224 w245] -> w219
                  disable-tunnel: [w223 w246] -> w218
                  disable-tunnel: w217 -> [w222 _]
                  frame Disabled {
                    n72 = Unbundle By Name(w226) -> ("FOV Rotation (deg)"=w227:dbl)
                    n73 = Not Equal?(x=w228, y=w227) -> (x != y?=w229:bool)
                    n74 = case shown="True" w229 {
                      tunnel: [w231 w232] -> w223
                      tunnel: w226 -> [w231 w238]
                      tunnel: w225 -> [w230 w237]
                      tunnel: [w230 w240] -> w224
                      tunnel: w228 -> [_ w235]
                      tunnel: w227 -> [_ w236]
                      tunnel: w222 -> [_ w234]
                      frame False {
                        # "mh: generovat warning ze cbk nastavuje reduntantne ?"
                      }
                      frame True {
                        n75 = call "SCMP CoMP-S Mechanism - rotation2.vi"("error in (no error)"=w237, "Auto Motors"=w234, "Old Rotation"=w236, "Desired Rotation"=w235) -> ("error out"=w239:errorcluster, "Rotation out"=w233:dbl)  [unwired: 6 in]
                        n76 = Bundle By Name(cluster=w238, "FOV Rotation (deg)"=w233) -> (w232:T4)
                        n77 = call "SCMP write init xml.vi"("error in (no error)"=w239, "FITS Header In"=w232) -> ("error out"=w240:errorcluster)  [unwired: 8 in, 1 out]
                      }
                    }
                  }
                  frame Enabled {
                    # "AISAS mech od v4.21\n(cez ASISAS class + COM port)"
                    n78 = Unbundle By Name(w248) -> ("Peripherals.AISAS Mech.lvclass"=w256:refnum<class "AISAS Mech.lvclass">)
                    n79 = To Variant(anything=w249) -> (Variant=w255:variant)
                    n80 = call "Write Move Motor.vi"("error in (no error)"=w247, "Desired Value"=w255, "Motor"=motor."Rotation", "AISAS Mech in"=w256) -> ("error out"=w252:errorcluster, "AISAS Mech out"=w251:refnum<class "AISAS Mech.lvclass">)  [unwired: 6 in]
                    n81 = call "Move.vi"("error in (no error)"=w252, "AISAS Mech in"=w251) -> ("error out"=w253:errorcluster, "AISAS Mech out"=w250:refnum<class "AISAS Mech.lvclass">, "status log"=w241:string)  [unwired: 7 in]
                    n82 = call "Read value.vi"("error in (no error)"=w253, "AISAS Mech in"=w250) -> ("error out"=w243:errorcluster, "Rotation"=w244:T17)  [unwired: 3 in, 5 out]
                    n83 = Bundle By Name(cluster=w248, "Peripherals.AISAS Mech.lvclass"=w250, "FOV Rotation (deg)"=w244) -> (w246:T4)
                    n84 = case shown="Error" w243 {
                      selector: w243 -> [w257 w260]
                      tunnel: [w257 w259] -> w242
                      tunnel: w241 -> [_ w258]
                      frame No Error {
                      }
                      frame Error {
                        n85 = call "SCMP - Write log v2.vi"("Error to log"=w260, "data"=w258) -> ("error out"=w259:errorcluster)  [unwired: 7 in, 2 out]
                      }
                    }
                    n86 = call "SCMP write init xml.vi"("error in (no error)"=w242, "FITS Header In"=w246) -> ("error out"=w245:errorcluster)  [unwired: 8 in, 1 out]
                  }
                }
              }
              frame "CAL-FW" {
                n87 = Decrement(x=w263) -> (x-1=w262:sgl)
                n88 = disable-structure shown="SCMP==COMP, Default" {
                  disable-tunnel: [w274 w279] -> w267
                  disable-tunnel: w266 -> [w273 w280]
                  disable-tunnel: w262 -> [w272 w281]
                  disable-tunnel: w265 -> [w271 w278]
                  disable-tunnel: [w270 w277] -> w264
                  disable-tunnel: w262 -> [w268 w275]
                  frame condition #0 {
                    n89 = Bundle By Name(cluster=w273, "SCD Calibration Optics"=w272) -> (w274:T4)
                    n90 = call "Optec IFW3 - Set Position with Error Handling.vi"("error in"=w271, "SCD Calibration Optics"=w268, "Filter Wheel Selector"=T16."Calibration Polarizers") -> ("error out"=w270:errorcluster)  [unwired: 6 in, 2 out]
                  }
                  frame condition #1 (active) {
                    n91 = Bundle By Name(cluster=w280, "COMP-S Calibration Wheel"=w281) -> (w279:T4)
                    n92 = call "CoMP-S Mechanism - FW.vi"("error in (no error)"=w278, "Calibration Polarizer Filters [Dark]"=w275, "Filter Wheel Selector"=T16."Calibration Polarizers") -> ("error out"=w277:errorcluster)  [unwired: 5 in, 3 out]
                  }
                }
              }
              frame "WAVELENGTH-FW" {
                n93 = Decrement(x=w284) -> (x-1=w283:sgl)
                n94 = disable-structure shown="SCMP==COMP, Default" {
                  disable-tunnel: w288 -> [w295 w301]
                  disable-tunnel: [w294 w300] -> w287
                  disable-tunnel: w283 -> [w293 w302]
                  disable-tunnel: w286 -> [w292 w299]
                  disable-tunnel: [w291 w298] -> w285
                  disable-tunnel: w283 -> [w290 w296]
                  frame condition #0 {
                    n95 = Bundle By Name(cluster=w295, "SCD Emission Line Filter"=w293) -> (w294:T4)
                    n96 = call "Optec IFW3 - Set Position with Error Handling.vi"("error in"=w292, "Emission Line Filter"=w290, "Filter Wheel Selector"=T16."Emission Line Filters") -> ("error out"=w291:errorcluster)  [unwired: 6 in, 2 out]
                  }
                  frame condition #1 (active) {
                    n97 = Bundle By Name(cluster=w301, "COMP-S Andover Filter Wheel"=w302) -> (w300:T4)
                    n98 = call "CoMP-S Mechanism - FW.vi"("error in (no error)"=w299, "Emission Line Filters [530.3 nm]"=w296, "Filter Wheel Selector"=T16."Emission Line Filters") -> ("error out"=w298:errorcluster)  [unwired: 5 in, 3 out]
                  }
                }
              }
              frame "DATATYPE" {
                n99 = disable-structure shown="Disabled" {
                  disable-tunnel: w305 -> [w310 w322]
                  disable-tunnel: [w309 w321] -> w304
                  frame Disabled {
                    n100 = case shown="9" w310 {
                      tunnel: [w311 w312 w313 w314 w315 w316 w317 w318 w319 w320] -> w309
                      frame 0, Default {
                        w311 = u16 0 items=["DARK", "FLAT", "CALI", "OBSE", "ABSO", "AURE", "TARG", "OBJE", "HOLE", "LIVE"] ("Data Type")
                      }
                      frame 1 {
                        w312 = u16 1 items=["DARK", "FLAT", "CALI", "OBSE", "ABSO", "AURE", "TARG", "OBJE", "HOLE", "LIVE"] ("Data Type")
                      }
                      frame 2 {
                        w313 = u16 2 items=["DARK", "FLAT", "CALI", "OBSE", "ABSO", "AURE", "TARG", "OBJE", "HOLE", "LIVE"] ("Data Type")
                      }
                      frame 3 {
                        w314 = u16 3 items=["DARK", "FLAT", "CALI", "OBSE", "ABSO", "AURE", "TARG", "OBJE", "HOLE", "LIVE"] ("Data Type")
                      }
                      frame 4 {
                        w315 = u16 4 items=["DARK", "FLAT", "CALI", "OBSE", "ABSO", "AURE", "TARG", "OBJE", "HOLE", "LIVE"] ("Data Type")
                      }
                      frame 5 {
                        w316 = u16 5 items=["DARK", "FLAT", "CALI", "OBSE", "ABSO", "AURE", "TARG", "OBJE", "HOLE", "LIVE"] ("Data Type")
                      }
                      frame 6 {
                        w317 = u16 6 items=["DARK", "FLAT", "CALI", "OBSE", "ABSO", "AURE", "TARG", "OBJE", "HOLE", "LIVE"] ("Data Type")
                      }
                      frame 7 {
                        w318 = u16 7 items=["DARK", "FLAT", "CALI", "OBSE", "ABSO", "AURE", "TARG", "OBJE", "HOLE", "LIVE"] ("Data Type")
                      }
                      frame 8 {
                        w319 = u16 8 items=["DARK", "FLAT", "CALI", "OBSE", "ABSO", "AURE", "TARG", "OBJE", "HOLE", "LIVE"] ("Data Type")
                      }
                      frame 9 {
                        w320 = u16 9 items=["DARK", "FLAT", "CALI", "OBSE", "ABSO", "AURE", "TARG", "OBJE", "HOLE", "LIVE"] ("Data Type")
                      }
                    }
                  }
                  frame Enabled {
                    n101 = To Unsigned Byte Integer(number=w322) -> (unsigned 8bit integer=w321:u8)
                  }
                }
                n102 = Bundle By Name(cluster=w307, "Data Type"=w304) -> (w306:T4)
              }
              frame "SET EXPOSURE" {
                # "mh jan2019\npre COMP je expozicia zadana v .rcp v [ms]\npre SCD je v [s] \n\nmaj2019\npre oba pristroje je v cbk v [ms]\n(andor sdk sa pracuje v sek)"
                n103 = Divide(x=w330, y=1000.0) -> (x/y=w326:dbl)
                n104 = for {
                  shift-right: [w339] -> w327
                  shift-left: w328 -> [w341]
                  tunnel: w324 -> [w335] mode=indexing
                  tunnel: w326 -> [w336]
                  tunnel: [w333] -> w325
                  tunnel: [w334] -> w323 mode=indexing
                  w338 = "ExposureTime" ("Feature")
                  n105 = Unbundle By Name(w335) -> ("Handle"=w337:i32)
                  n106 = call <userlib>:"AT Set Float A.vi"("error in (no error)"=w341, "Value"=w336, "Feature"=w338, "Hndl"=w337) -> ("error out"=w340:errorcluster)  [unwired: 6 in, 1 out]
                  n107 = call <userlib>:"AT Get Float A.vi"("error in (no error)"=w340, "Feature"=w338, "Handle"=w337) -> ("error out"=w339:errorcluster, "Value"=w333:dbl)  [unwired: 6 in, 1 out]
                  n108 = Bundle By Name(cluster=w335, "Exposure (s)"=w333) -> (w334:T1)
                }
                "Exposure (s)" <- w325
                n109 = Bundle By Name(cluster=w332, "Exposure (s)"=w325) -> (w331:T4)
              }
              frame "CBK COMMENTS" {
                n110 = call "SCMP - Write log v2.vi"("Error to log"=w346, "data"=w344) -> ("error out"=w345:errorcluster)  [unwired: 7 in, 2 out]
              }
              frame "MOVE-PI" {
                n111 = Unbundle By Name(w348) -> ("Peripherals.PI Stages"=w347:bool)
                n112 = case shown="True" w347 {
                  tunnel: w348 -> [w355 w368]
                  tunnel: [w355 w367] -> w354
                  tunnel: w353 -> [_ w366]
                  tunnel: [w356 w365] -> w352
                  tunnel: w351 -> [w356 w364]
                  tunnel: w350 -> [_ w359]
                  frame False {
                  }
                  frame True {
                    w358 = sgl -1000.0 ("element")
                    n113 = Number To Boolean Array(number=w366) -> (Boolean array=w363:bool[])
                    "Changes 0 or 1 to true/false for absolute or relative control 2" <- w363
                    n114 = Index Array(array=w363, index=0) -> (element=w361:bool)
                    n115 = Build Array(w359, w358, w358) -> (w357:sgl[])
                    n116 = call "SCMP - Control PI Stage Position2.vi"("error in"=w364, "Absolute (F) or \nRelative (T) Move"=w361, "set values"=w357) -> ("error out"=w365:errorcluster, "Position"=w360:dbl[])  [unwired: 6 in, 1 out]
                    n117 = Bundle By Name(cluster=w368, "Camera PI (mm)"=w360) -> (w367:T4)
                  }
                }
              }
              frame "MOVE-PI2" {
                n118 = Unbundle By Name(w370) -> ("Peripherals.PI Stages"=w369:bool)
                n119 = case shown="True" w369 {
                  tunnel: w370 -> [w377 w390]
                  tunnel: [w377 w389] -> w376
                  tunnel: w375 -> [_ w388]
                  tunnel: [w378 w387] -> w374
                  tunnel: w373 -> [w378 w386]
                  tunnel: w372 -> [_ w379]
                  frame False {
                  }
                  frame True {
                    w380 = sgl -1000.0 ("element")
                    n120 = Number To Boolean Array(number=w388) -> (Boolean array=w385:bool[])
                    "Changes 0 or 1 to true/false for absolute or relative control 3" <- w385
                    n121 = Index Array(array=w385, index=0) -> (element=w383:bool)
                    n122 = Build Array(w380, w379, w380) -> (w381:sgl[])
                    n123 = call "SCMP - Control PI Stage Position2.vi"("error in"=w386, "Absolute (F) or \nRelative (T) Move"=w383, "set values"=w381) -> ("error out"=w387:errorcluster, "Position"=w382:dbl[])  [unwired: 6 in, 1 out]
                    n124 = Bundle By Name(cluster=w390, "Camera PI (mm)"=w382) -> (w389:T4)
                  }
                }
              }
              frame "MOVE-PI3" {
                n125 = Unbundle By Name(w392) -> ("Peripherals.PI Stages"=w391:bool)
                n126 = case shown="True" w391 {
                  tunnel: w392 -> [w399 w412]
                  tunnel: [w399 w411] -> w398
                  tunnel: w397 -> [_ w410]
                  tunnel: [w400 w409] -> w396
                  tunnel: w395 -> [w400 w408]
                  tunnel: w394 -> [_ w401]
                  frame False {
                  }
                  frame True {
                    w402 = sgl -1000.0 ("element")
                    n127 = Number To Boolean Array(number=w410) -> (Boolean array=w407:bool[])
                    "Changes 0 or 1 to true/false for absolute or relative control 4" <- w407
                    n128 = Index Array(array=w407, index=0) -> (element=w405:bool)
                    n129 = Build Array(w402, w402, w401) -> (w403:sgl[])
                    n130 = call "SCMP - Control PI Stage Position2.vi"("error in"=w408, "Absolute (F) or \nRelative (T) Move"=w405, "set values"=w403) -> ("error out"=w409:errorcluster, "Position"=w404:dbl[])  [unwired: 6 in, 1 out]
                    n131 = Bundle By Name(cluster=w412, "Camera PI (mm)"=w404) -> (w411:T4)
                  }
                }
              }
              frame "DWELL TIME" {
                n132 = call "SCMP - Run Cbk dwell time.vi"("error in (no error)"=w417, "Dwell time [s]"=w416) -> ("error out"=w414:errorcluster, "Aborted?"=w415:bool)  [unwired: 8 in]
                n133 = case shown="True" w415 {
                  tunnel: [w420 w422] -> w413
                  tunnel: w414 -> [w420 w423]
                  frame False {
                  }
                  frame True {
                    # "dwell time aborted"
                    n134 = Unbundle By Name(w423) -> ("source"=w421:string)
                    n135 = call "SCMP - Write log v2.vi"("Error to log"=w423, "data"=w421) -> ("error out"=w422:errorcluster)  [unwired: 7 in, 2 out]
                  }
                }
              }
            }
          }
          frame Error {
          }
        }
        n136 = Unbundle By Name(w30) -> ("status"=w32:bool)
        n137 = Or(x=w32, y="Stop Cookbook") -> (x .or. y?=w29:bool)
      }
      n138 = global read "Globals.vi" "SCMP"() -> (w10:enum16{"COMP", "SCD"})
      n139 = case shown="\"COMP\", Default" w10 {
        tunnel: w13 -> [w24 w28]
        tunnel: [w23 w26] -> w11
        frame "COMP", Default {
          n140 = Unbundle By Name(w24) -> ("COMP-S Andover Filter Wheel"=w25:T9)
          n141 = call "COMP - wavelenght.vi"("COMP-S Andover Filter Wheel"=w25) -> ("Wavelength (nm)"=w23:dbl)  [unwired: 10 in]
        }
        frame "SCD" {
          n142 = Unbundle By Name(w28) -> ("SCD Emission Line Filter"=w27:T7)
          n143 = call "SCD - wavelenght.vi"("SCD Emission Line Filter"=w27) -> ("Numeric"=w26:dbl)  [unwired: 10 in]
        }
      }
      n144 = Bundle By Name(cluster=w13, "Wavelength (nm)"=w11) -> (w12:T4)
    }
    frame Error {
    }
  }
  "Error out" <- w8
  "Updated Header" <- w1
  n145 = case shown="True" w6 {
    tunnel: ["Cookbook Completed" ("data") "Cookbook Interrupted" ("data")] -> w7
    frame False {
    }
    frame True {
    }
  }
  "Result" <- w7
